vi "Create Channel Defaults Array.vi"(8 "error in":errorcluster, 11 "Electronic Load in":refnum<class "Electronic Load.lvclass">) -> (0 "error out":errorcluster, 3 "Electronic Load out":refnum<class "Electronic Load.lvclass">)   [LabVIEW 2019, in "Electronic Load.lvlib" / "Electronic Load.lvclass"]
uses:
  Library/Electronic Load.lvclass
  Library/Electronic Load.lvclass/Electronic Load.ctl
  Custom Controls/Trigger Settings.ctl
  Custom Controls/E-Load Mode.ctl
  Custom Controls/OCP Settings.ctl
  Custom Controls/E-Load Function.ctl
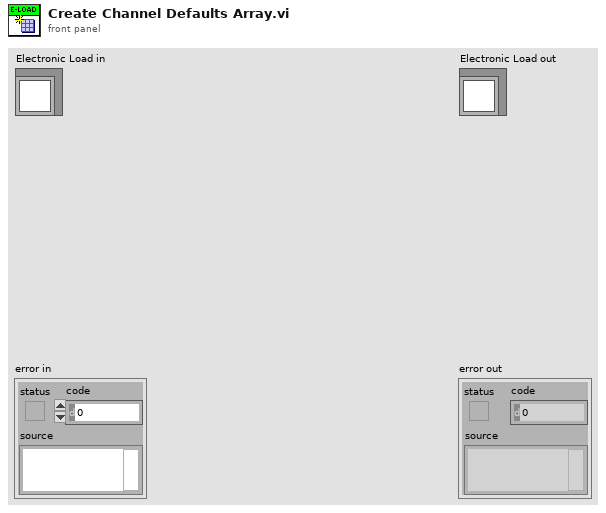
[diagram p1: front panel]
types:
  T1 = typedef "Electronic Load.lvlib/Electronic Load.lvclass/Trigger Settings.ctl" = cluster{"Mode":T2, "Initial":dbl, "Transient":dbl, "Interval":dbl, "Width":dbl, "Delay":dbl, "Data Pts":i32, "Slew Rate":dbl}
  T2 = typedef "Electronic Load.lvlib/Electronic Load.lvclass/E-Load Mode.ctl" = enum16{"Current", "Resistance", "Voltage"}
  T3 = typedef "Electronic Load.lvlib/Electronic Load.lvclass/E-Load Function.ctl" = cluster{"Mode":T2, "Input Level":dbl, "Output":bool, "Slew Rate":dbl}
  T4 = typedef "Electronic Load.lvlib/Electronic Load.lvclass/OCP Settings.ctl" = cluster{"OCP_Enabled":bool, "OCP Level":dbl, "OCP Delay":dbl}
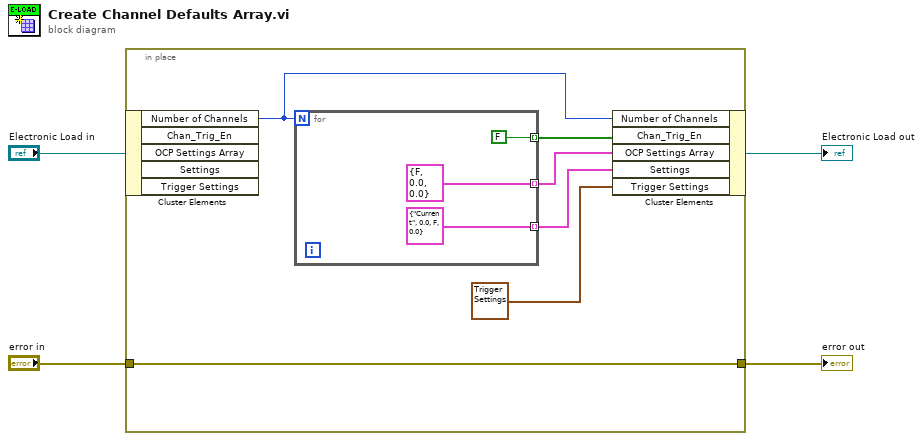
[diagram p0: block diagram]
diagram:
  n1 = in-place {
    in-place-border: "error in" -> [w10]
    in-place-border: [w10] -> w2
    n2 = in-place-cluster #1("Electronic Load in") -> ("Number of Channels"=w9:i32)  [unwired: 4 out]
    n3 = for {
      N: w9 -> [_]
      tunnel: [T4 {"OCP_Enabled"=FALSE, "OCP Level"=0.0, "OCP Delay"=0.0} ("OCP Settings")] -> w8 mode=indexing
      tunnel: [T3 {"Mode"=enum."Current", "Input Level"=0.0, "Output"=FALSE, "Slew Rate"=0.0} ("Function")] -> w7 mode=indexing
      tunnel: [FALSE] -> w5 mode=indexing
    }
    n4 = in-place-cluster #1("Number of Channels"=w9, "Chan_Trig_En"=w5, "OCP Settings Array"=w8, "Settings"=w7, "Trigger Settings"=T1 {"Mode"=enum."Current", "Initial"=0.0, "Transient"=0.0, "Interval"=0.0, "Width"=0.0, "Delay"=0.0, "Data Pts"=0, "Slew Rate"=15000.0}) -> (→"Electronic Load out":refnum<class "Electronic Load.lvclass">)
  }
  "error out" <- w2
